vi "delay.vi"(8 "error in (no error)":errorcluster, 9 "enable":bool=TRUE, 10 "Multiplier":i32=1, 11 "milliseconds to wait":u32) -> (0 "error out (no error)":errorcluster, 3 "TimeOut":bool)   [LabVIEW 2018]
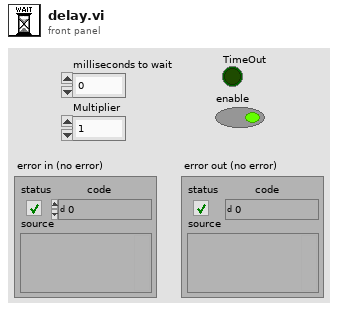
[diagram p1: front panel]
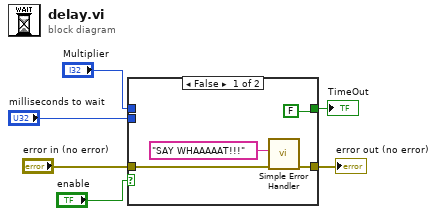
[diagram p0: block diagram]
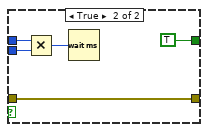
[diagram p2: hidden frame]
diagram:
  n1 = case shown="False" "enable" {
    tunnel: "milliseconds to wait" -> [_ w14]
    tunnel: "Multiplier" -> [_ w15]
    tunnel: "error in (no error)" -> [w9 w12]
    tunnel: [w10 w12] -> w2
    tunnel: [FALSE TRUE] -> w1
    frame False {
      n2 = call <vilib>:"Simple Error Handler.vi"("error source (\" \")"="SAY WHAAAAAT!!!" ("error source (\" \")"), "error in (no error)"=w9) -> ("error out"=w10:errorcluster)  [unwired: 3 in, 4 out]
    }
    frame True {
      n3 = Multiply(x=w15, y=w14) -> (x*y=w13:u32)
      n4 = Wait (ms)(milliseconds to wait=w13) -> ()  [unwired: 1 out]
    }
  }
  "error out (no error)" <- w2
  "TimeOut" <- w1
